vi "Receive Single U32 CMD and String Data.vi"(0 "TCP Ref In":refnum<k5>, 1 "Time Out(ms)":i32=100, 11 "error in (no error)":errorcluster) -> (4 "TCP Ref Out":refnum<k5>, 6 "CMD":u32, 8 "Data":string, 15 "error out":errorcluster)   [LabVIEW 2024]
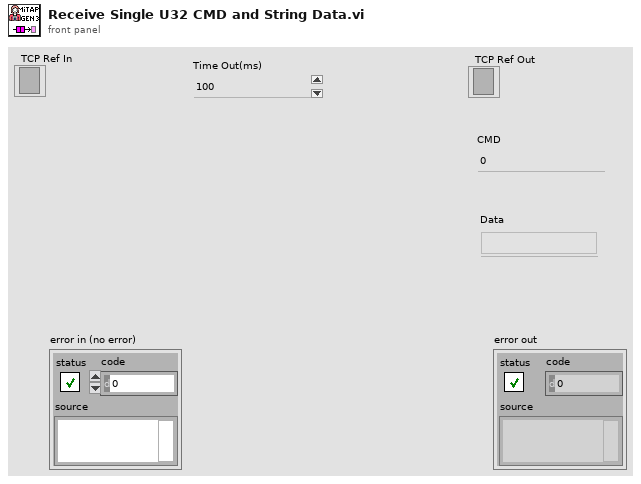
[diagram p1: front panel]
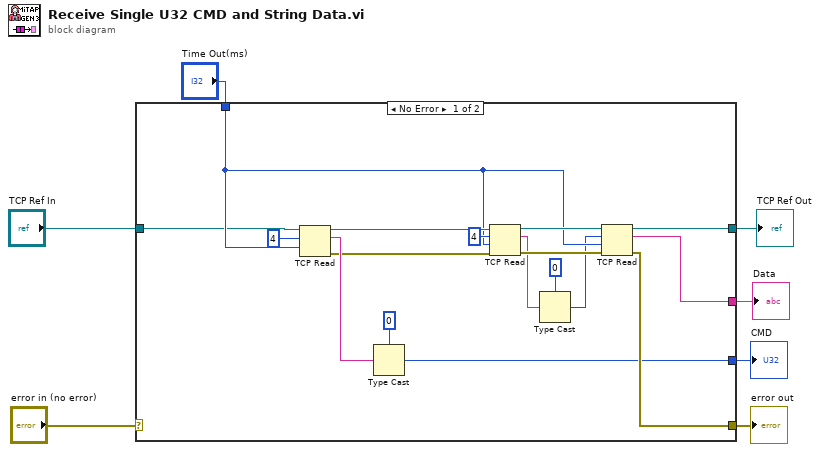
[diagram p0: block diagram]
diagram:
  n1 = case shown="No Error" "error in (no error)" {
    selector: "error in (no error)" -> [_ w26]
    tunnel: [w14 w26] -> w6
    tunnel: [w13 _] -> w5
    tunnel: [w12 _] -> w4
    tunnel: "Time Out(ms)" -> [w11 _]
    tunnel: "TCP Ref In" -> [w10 w25]
    tunnel: [w9 w25] -> w1
    frame No Error {
      n2 = TCP Read(connection ID=w10, bytes to read=4, 9:w11) -> (connection ID out=w23:refnum<k5>, data out=w22:string, error out=w20:errorcluster)  [unwired: 2 in]
      n3 = Type Cast(type=u32 0 ("bytes to read"), x=w22) -> (*(type *) &x=w13:u32)
      n4 = TCP Read(connection ID=w23, bytes to read=4, error in (no error)=w20, 9:w11) -> (connection ID out=w17:refnum<k5>, data out=w15:string, error out=w18:errorcluster)  [unwired: 1 in]
      n5 = Type Cast(type=0 ("bytes to read"), x=w15) -> (*(type *) &x=w8:i32)
      n6 = TCP Read(connection ID=w17, bytes to read=w8, error in (no error)=w18, 9:w11) -> (connection ID out=w9:refnum<k5>, data out=w12:string, error out=w14:errorcluster)  [unwired: 1 in]
    }
    frame Error {
    }
  }
  "error out" <- w6
  "CMD" <- w5
  "Data" <- w4
  "TCP Ref Out" <- w1
